vi "GetSectionMap.vi"(8 "error in (no error)":errorcluster caption="에러 입력(에러 없음)", 10 "Section":T2(ring)=enum."DataSection", 11 "ABFFIO 입력":refnum<class "ABFFIO.lvclass">) -> (0 "error out":errorcluster caption="에러 출력", 2 "SectionMap":T1, 3 "ABFFIO 출력":refnum<class "ABFFIO.lvclass">)   [LabVIEW 2017, in "ABFFIO.lvclass"]
uses:
  ABFFIO.lvclass
  ABFFIO.lvclass/ABFFIO.ctl
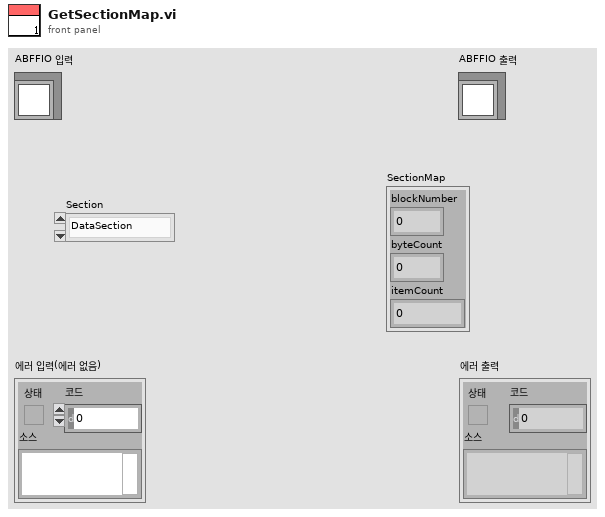
[diagram p1: front panel]
types:
  T1 = cluster{"blockNumber":u32, "byteCount":u32, "itemCount":u32}
  T2 = enum16{"ProtocolSection", "ADCSection", "DACSection", "EpochSection", "ADCPerDACSection", "EpochPerDACSection", "StringsSection", "DataSection", "TagSection"}
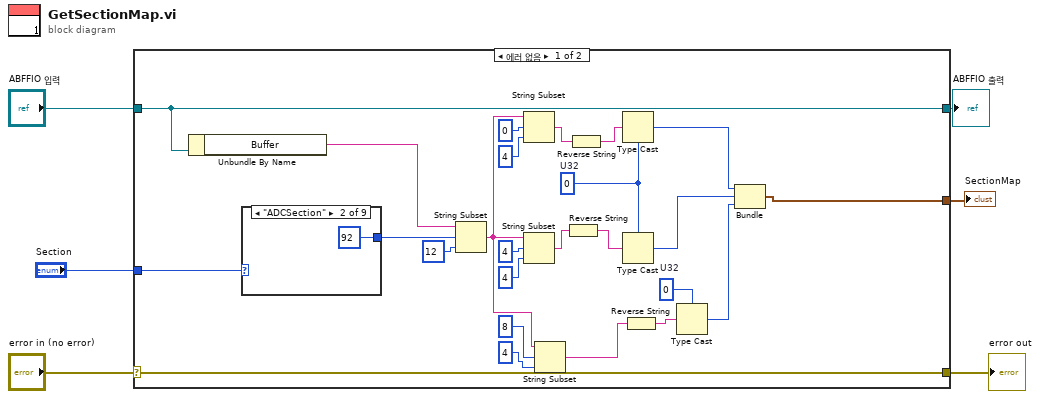
[diagram p0: block diagram]
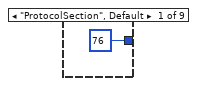
[diagram p2: hidden frame]
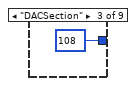
[diagram p3: hidden frame]
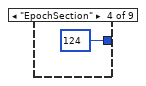
[diagram p4: hidden frame]
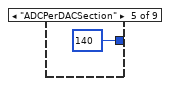
[diagram p5: hidden frame]
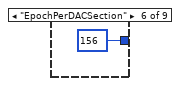
[diagram p6: hidden frame]
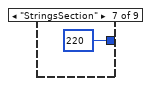
[diagram p7: hidden frame]
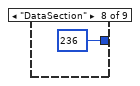
[diagram p8: hidden frame]
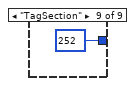
[diagram p9: hidden frame]
diagram:
  n1 = case shown="에러 없음" "error in (no error)" {
    selector: "error in (no error)" -> [w31 w42]
    tunnel: [w31 w42] -> w5
    tunnel: [w13 w41] -> w3
    tunnel: "ABFFIO 입력" -> [w13 w41]
    tunnel: "Section" -> [w14 _]
    tunnel: [w11 _] -> w1
    frame No Error {
      w22 = u32 0  # U32
      w21 = u32 0  # U32
      n2 = Unbundle By Name(w13) -> ("Buffer"=w12:string)
      n3 = case shown="\"ADCSection\"" w14 {
        tunnel: [76 92 ("오프셋(0)") 108 124 140 156 220 236 252] -> w15
        frame "ProtocolSection", Default {
        }
        frame "ADCSection" {
        }
        frame "DACSection" {
        }
        frame "EpochSection" {
        }
        frame "ADCPerDACSection" {
        }
        frame "EpochPerDACSection" {
        }
        frame "StringsSection" {
        }
        frame "DataSection" {
        }
        frame "TagSection" {
        }
      }
      n4 = String Subset(string=w12, offset (0)=w15, length (rest)=12 ("길이(나머지)")) -> (substring=w27:string)
      n5 = String Subset(string=w27, offset (0)=0 ("오프셋(0)"), length (rest)=4 ("길이(나머지)")) -> (substring=w8:string)
      n6 = String Subset(string=w27, offset (0)=4 ("오프셋(0)"), length (rest)=4 ("길이(나머지)")) -> (substring=w10:string)
      n7 = String Subset(string=w27, offset (0)=8 ("오프셋(0)"), length (rest)=4 ("길이(나머지)")) -> (substring=w30:string)
      n8 = Reverse String(1:w10) -> (0:w9:string)
      n9 = Reverse String(1:w8) -> (0:w7:string)
      n10 = Type Cast(type=w21, x=w7) -> (*(type *) &x=w24:u32)
      n11 = Type Cast(type=w21, x=w9) -> (*(type *) &x=w25:u32)
      n12 = Reverse String(1:w30) -> (0:w23:string)
      n13 = Type Cast(type=w22, x=w23) -> (*(type *) &x=w26:u32)
      n14 = Bundle("U32"=w24, "U32"=w25, "U32"=w26) -> (w11:cluster{"U32":u32, "U32":u32, "U32":u32})  [unwired: 1 in]
    }
    frame Error {
    }
  }
  "error out" <- w5
  "ABFFIO 출력" <- w3
  "SectionMap" <- w1
